vi "Convert from XML Children.vi"(8 "error in":errorcluster, 11 "KA string":string="<DB_Connection>c:\\temp</DB_Connection>") -> (0 "error out":errorcluster, 3 "keyed array":T1)   [LabVIEW 2012, in "Car Wash.lvlib" / "Tools_KeyedArray.lvlib"]
uses:
  Tools_KeyedArray.lvlib
  KeyedArray.ctl
  Map String.vi
  String/Get Case Matching.vi
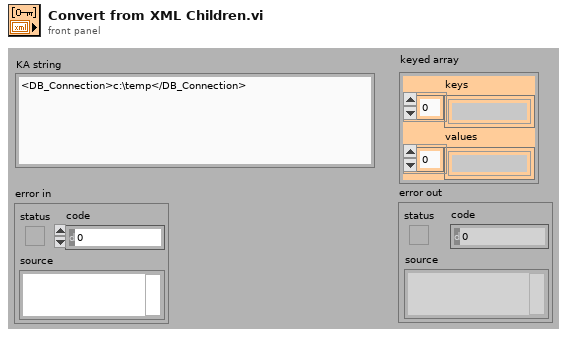
[diagram p1: front panel]
types:
  T1 = typedef "Car Wash.lvlib/Tools_KeyedArray.lvlib/KeyedArray.ctl" = cluster{"keys":string[], "values":string[]}
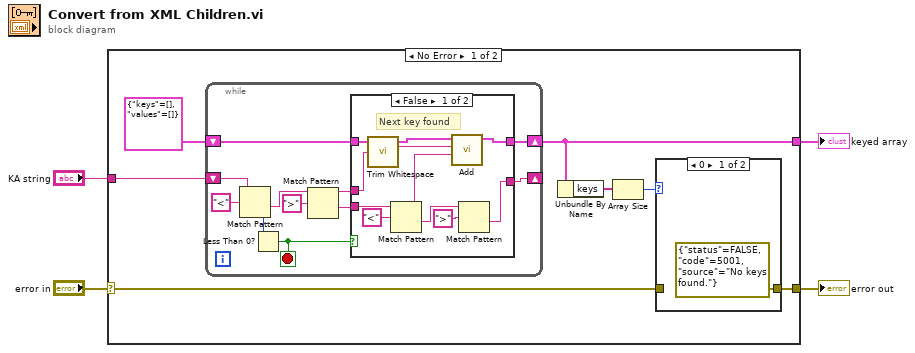
[diagram p0: block diagram]
diagram:
  n1 = case shown="No Error" "error in" {
    selector: "error in" -> [w5 w37]
    tunnel: [w8 w37] -> w3
    tunnel: [w7 _] -> w2
    tunnel: "KA string" -> [w6 _]
    frame No Error {
      n2 = while {
        shift-right: [w18] -> _
        shift-left: w6 -> [w24]
        shift-right: [w19] -> w7
        shift-left: T1 {"keys"=[], "values"=[]} ("keyed array") -> [w20]
        stop <- w21 stop-if-true
        n3 = Match Pattern(string=w24, regular expression="<") -> (after substring=w17:string, offset past match=w22:i32)  [unwired: 3 out]
        n4 = Less Than 0?(x=w22) -> (x < 0?=w21:bool)
        n5 = Match Pattern(string=w17, regular expression=">") -> (before substring=w15:string, after substring=w14:string)  [unwired: 3 out]
        n6 = case shown="False" w21 {
          tunnel: w15 -> [w34 _]
          tunnel: w20 -> [w33 w36]
          tunnel: [w32 w36] -> w19
          tunnel: w14 -> [w25 w35]
          tunnel: [w27 w35] -> w18
          frame False {
            # "Next key found"
            n7 = call <vilib>:"Trim Whitespace.vi"("string"=w34) -> ("trimmed string"=w31:string)  [unwired: 1 in]
            n8 = Match Pattern(string=w25, regular expression="<") -> (before substring=w26:string, after substring=w29:string)  [unwired: 3 out]
            n9 = call "Add.vi"("value"=w26, "key"=w31, "array in"=w33) -> ("array out"=w32:T1)  [unwired: 1 in, 3 out]
            n10 = Match Pattern(string=w29, regular expression=">") -> (after substring=w27:string)  [unwired: 4 out]
          }
          frame True {
            # "No key found"
          }
        }
      }
      n11 = Unbundle By Name(w7) -> ("keys"=w10:string[])
      n12 = Array Size(array=w10) -> (size(s)=w9:i32)
      n13 = case shown="0" w9 {
        tunnel: [errorcluster {"status"=FALSE, "code"=5001, "source"="No keys found."} ("error IO") w13] -> w8
        tunnel: w5 -> [_ w13]
        frame 0 {
        }
        frame 1, Default {
        }
      }
    }
    frame Error {
    }
  }
  "error out" <- w3
  "keyed array" <- w2
